vi "test json to variant int.vi"(8 "error in (no error)":errorcluster) -> (0 "error out":errorcluster)   [LabVIEW 2019, in "labview_json_tests.lvlib"]
uses:
  labview_json_tests.lvlib
  lib/labview_json.lvlib
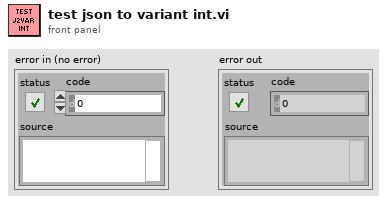
[diagram p1: front panel]
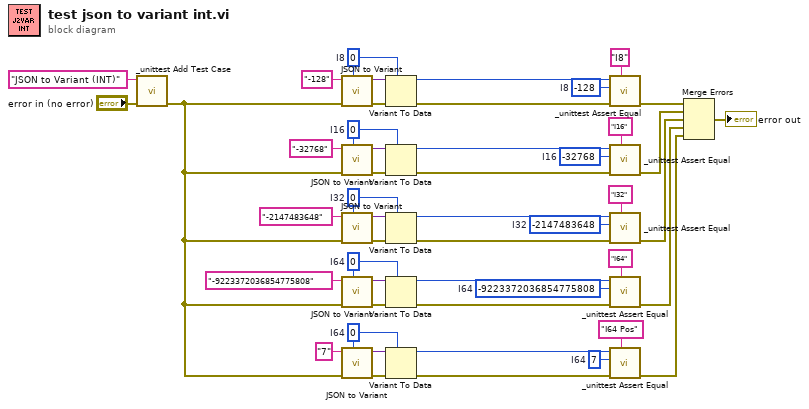
[diagram p0: block diagram]
diagram:
  w26 = i64 7  # I64
  w15 = i64 0  # I64
  w29 = i64 -9223372036854775808  # I64
  w14 = i64 0  # I64
  w36 = -2147483648  # I32
  w13 = 0  # I32
  w37 = i16 -32768  # I16
  w12 = i16 0  # I16
  w38 = i8 -128  # I8
  w11 = i8 0  # I8
  n1 = call "_unittest Add Test Case.vi"("error in (no error)"="error in (no error)", "Test Case"="JSON to Variant (INT)") -> ("error out"=w21:errorcluster)  [unwired: 9 in]
  n2 = call "JSON to Variant.vi"("Variant Type"=w11, "error in (no error)"=w21, "JSON"="-128") -> ("error out"=w44:errorcluster, "Variant out"=w10:variant)  [unwired: 7 in]
  n3 = call "JSON to Variant.vi"("Variant Type"=w12, "error in (no error)"=w21, "JSON"="-32768") -> ("error out"=w41:errorcluster, "Variant out"=w9:variant)  [unwired: 7 in]
  n4 = call "JSON to Variant.vi"("Variant Type"=w13, "error in (no error)"=w21, "JSON"="-2147483648") -> ("error out"=w34:errorcluster, "Variant out"=w8:variant)  [unwired: 7 in]
  n5 = call "JSON to Variant.vi"("Variant Type"=w14, "error in (no error)"=w21, "JSON"="-9223372036854775808") -> ("error out"=w31:errorcluster, "Variant out"=w7:variant)  [unwired: 7 in]
  n6 = call "JSON to Variant.vi"("Variant Type"=w15, "error in (no error)"=w21, "JSON"="7") -> ("error out"=w24:errorcluster, "Variant out"=w6:variant)  [unwired: 7 in]
  n7 = Variant To Data(error in=w44, type=w11, Variant=w10) -> (data=w1:i8, error out=w16:errorcluster)
  n8 = Variant To Data(error in=w41, type=w12, Variant=w9) -> (data=w2:i16, error out=w17:errorcluster)
  n9 = Variant To Data(error in=w34, type=w13, Variant=w8) -> (data=w3:i32, error out=w18:errorcluster)
  n10 = Variant To Data(error in=w31, type=w14, Variant=w7) -> (data=w4:i64, error out=w19:errorcluster)
  n11 = Variant To Data(error in=w24, type=w15, Variant=w6) -> (data=w5:i64, error out=w20:errorcluster)
  n12 = call "_unittest Assert Equal.vi"("Message"="I8", "error in (no error)"=w16, "Expected Value"=w38, "Actual Value"=w1) -> ("error out"=w47:errorcluster)  [unwired: 7 in]
  n13 = call "_unittest Assert Equal.vi"("Message"="I16", "error in (no error)"=w17, "Expected Value"=w37, "Actual Value"=w2) -> ("error out"=w39:errorcluster)  [unwired: 7 in]
  n14 = call "_unittest Assert Equal.vi"("Message"="I32", "error in (no error)"=w18, "Expected Value"=w36, "Actual Value"=w3) -> ("error out"=w28:errorcluster)  [unwired: 7 in]
  n15 = call "_unittest Assert Equal.vi"("Message"="I64", "error in (no error)"=w19, "Expected Value"=w29, "Actual Value"=w4) -> ("error out"=w27:errorcluster)  [unwired: 7 in]
  n16 = call "_unittest Assert Equal.vi"("Message"="I64 Pos", "error in (no error)"=w20, "Expected Value"=w26, "Actual Value"=w5) -> ("error out"=w22:errorcluster)  [unwired: 7 in]
  n17 = Merge Errors(w47, w39, w28, w27, w22) -> (→"error out":errorcluster)
